vi "Check Data Model.vi"(8 "error in":errorcluster, 11 "device data model in":refnum<class "Standard Data Model.lvclass">) -> (0 "error out":errorcluster, 3 "device data model out":refnum<class "Standard Data Model.lvclass">)   [LabVIEW 2012, in "Standard Data Model.lvclass"]
doc: "This VI ensures that the data model has at least 65,535 values of every type. This is required for certain modbus function codes."
uses:
  Standard Data Model.lvclass
  Standard Data Model.lvclass/Standard Data Model.ctl
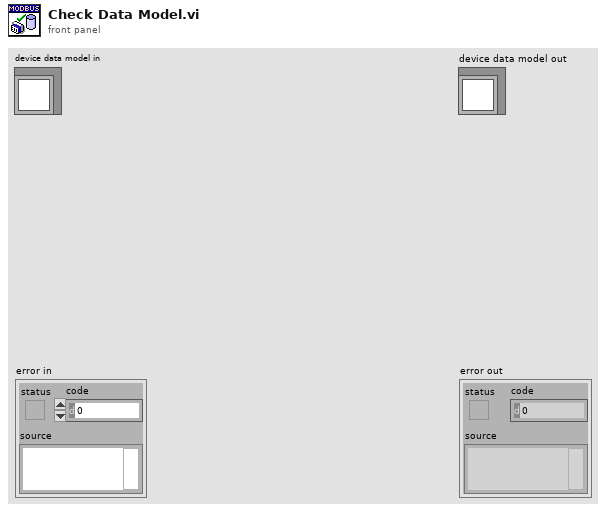
[diagram p1: front panel]
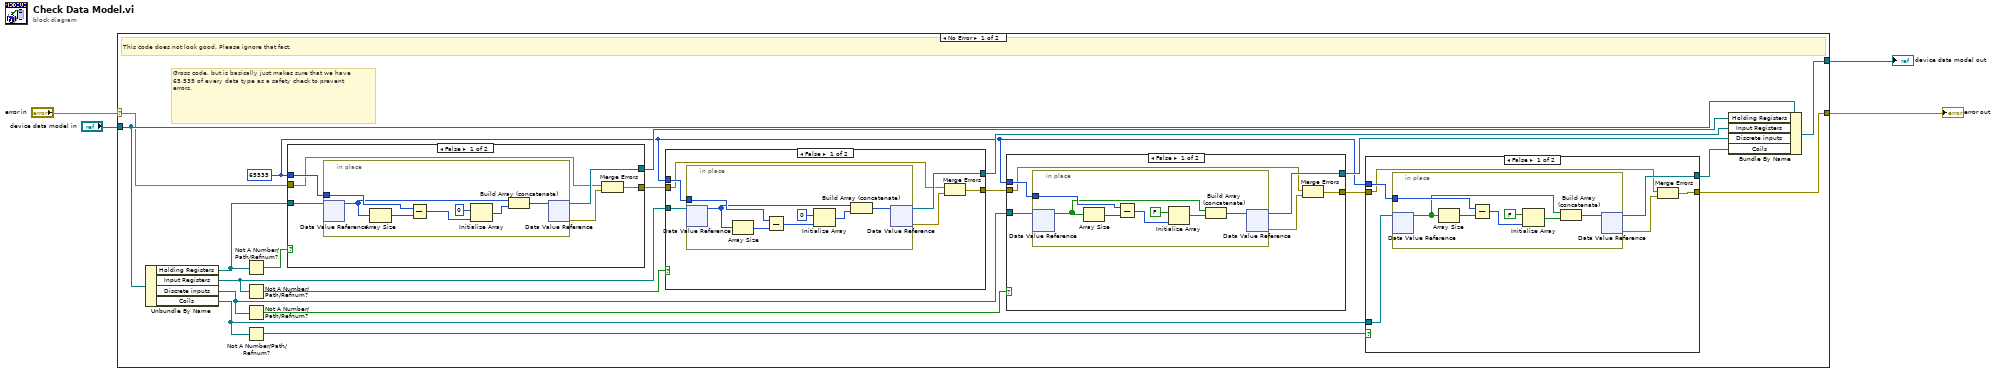
[diagram p0: block diagram]
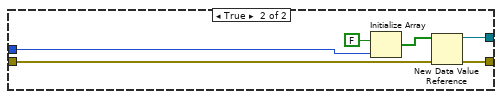
[diagram p2: hidden frame]
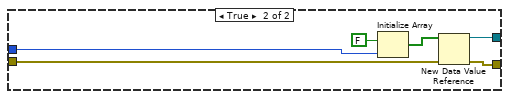
[diagram p3: hidden frame]
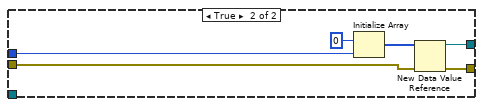
[diagram p4: hidden frame]
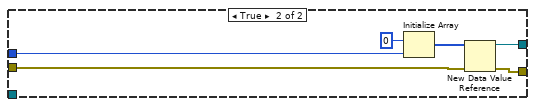
[diagram p5: hidden frame]
diagram:
  n1 = case shown="No Error" "error in" {
    selector: "error in" -> [w5 w102]
    tunnel: "device data model in" -> [w19 w101]
    tunnel: [w18 w101] -> w3
    tunnel: [w9 w102] -> w2
    frame No Error {
      w6 = u16 65535 ("x")
      # "Gross code, but is basically just makes sure that we have 65,535 of every data type as a safety check to prevent errors."
      # "This code does not look good. Please ignore that fact."
      n2 = Unbundle By Name(w19) -> ("Holding Registers"=w23:refnum<data-value>, "Input Registers"=w21:refnum<data-value>, "Discrete inputs"=w14:refnum<data-value>, "Coils"=w7:refnum<data-value>)
      n3 = Not A Number/Path/Refnum?(number/path/refnum=w23) -> (NaN/Path/Refnum?=w24:bool)
      n4 = Not A Number/Path/Refnum?(number/path/refnum=w21) -> (NaN/Path/Refnum?=w22:bool)
      n5 = Not A Number/Path/Refnum?(number/path/refnum=w14) -> (NaN/Path/Refnum?=w15:bool)
      n6 = Not A Number/Path/Refnum?(number/path/refnum=w7) -> (NaN/Path/Refnum?=w11:bool)
      n7 = case shown="False" w24 {
        tunnel: w5 -> [w82 w99]
        tunnel: [w84 w97] -> w17
        tunnel: [w85 w96] -> w20
        tunnel: w23 -> [w86 _]
        tunnel: w6 -> [w83 w95]
        frame False {
          n8 = in-place {
            in-place-border: w83 -> [w94]
            n9 = in-place-dvr #1(w86) -> (w90:u16[])  [unwired: 1 out]
            n10 = Array Size(array=w90) -> (size(s)=w93:i32)
            n11 = Subtract(x=w94, y=w93) -> (x-y=w92:i32)
            n12 = Initialize Array(u16 0 ("element"), w92) -> (w89:u16[])
            n13 = Build Array (concatenate)(w90, w89) -> (w88:u16[])
            n14 = in-place-dvr #1(w88) -> (w84:refnum<data-value>, w87:errorcluster)
          }
          n15 = Merge Errors(w82, w87) -> (w85:errorcluster)
        }
        frame True {
          n16 = Initialize Array(u16 0 ("element"), w95) -> (w98:u16[])
          n17 = New Data Value Reference(data value=w98, error in=w99) -> (data value reference=w97:refnum<data-value>, error out=w96:errorcluster)
        }
      }
      n18 = case shown="False" w22 {
        tunnel: w20 -> [w63 w80]
        tunnel: [w65 w78] -> w16
        tunnel: [w66 w77] -> w12
        tunnel: w21 -> [w67 _]
        tunnel: w6 -> [w64 w76]
        frame False {
          n19 = in-place {
            in-place-border: w64 -> [w75]
            n20 = in-place-dvr #2(w67) -> (w71:u16[])  [unwired: 1 out]
            n21 = Array Size(array=w71) -> (size(s)=w74:i32)
            n22 = Subtract(x=w75, y=w74) -> (x-y=w73:i32)
            n23 = Initialize Array(u16 0 ("element"), w73) -> (w70:u16[])
            n24 = Build Array (concatenate)(w71, w70) -> (w69:u16[])
            n25 = in-place-dvr #2(w69) -> (w65:refnum<data-value>, w68:errorcluster)
          }
          n26 = Merge Errors(w63, w68) -> (w66:errorcluster)
        }
        frame True {
          n27 = Initialize Array(u16 0 ("element"), w76) -> (w79:u16[])
          n28 = New Data Value Reference(data value=w79, error in=w80) -> (data value reference=w78:refnum<data-value>, error out=w77:errorcluster)
        }
      }
      n29 = case shown="False" w15 {
        tunnel: w12 -> [w44 w62]
        tunnel: [w46 w57] -> w13
        tunnel: [w47 w60] -> w8
        tunnel: w14 -> [w48 _]
        tunnel: w6 -> [w45 w59]
        frame False {
          n30 = in-place {
            in-place-border: w45 -> [w56]
            n31 = in-place-dvr #3(w48) -> (w52:bool[])  [unwired: 1 out]
            n32 = Array Size(array=w52) -> (size(s)=w55:i32)
            n33 = Subtract(x=w56, y=w55) -> (x-y=w54:i32)
            n34 = Initialize Array(FALSE, w54) -> (w51:bool[])
            n35 = Build Array (concatenate)(w52, w51) -> (w50:bool[])
            n36 = in-place-dvr #3(w50) -> (w46:refnum<data-value>, w49:errorcluster)
          }
          n37 = Merge Errors(w44, w49) -> (w47:errorcluster)
        }
        frame True {
          n38 = Initialize Array(FALSE, w59) -> (w61:bool[])
          n39 = New Data Value Reference(data value=w61, error in=w62) -> (data value reference=w57:refnum<data-value>, error out=w60:errorcluster)
        }
      }
      n40 = case shown="False" w11 {
        tunnel: w8 -> [w25 w43]
        tunnel: [w27 w39] -> w10
        tunnel: [w28 w41] -> w9
        tunnel: w7 -> [w29 _]
        tunnel: w6 -> [w26 w40]
        frame False {
          n41 = in-place {
            in-place-border: w26 -> [w37]
            n42 = in-place-dvr #4(w29) -> (w33:bool[])  [unwired: 1 out]
            n43 = Array Size(array=w33) -> (size(s)=w36:i32)
            n44 = Subtract(x=w37, y=w36) -> (x-y=w35:i32)
            n45 = Initialize Array(FALSE, w35) -> (w32:bool[])
            n46 = Build Array (concatenate)(w33, w32) -> (w31:bool[])
            n47 = in-place-dvr #4(w31) -> (w27:refnum<data-value>, w30:errorcluster)
          }
          n48 = Merge Errors(w25, w30) -> (w28:errorcluster)
        }
        frame True {
          n49 = Initialize Array(FALSE, w40) -> (w42:bool[])
          n50 = New Data Value Reference(data value=w42, error in=w43) -> (data value reference=w39:refnum<data-value>, error out=w41:errorcluster)
        }
      }
      n51 = Bundle By Name(cluster=w19, "Holding Registers"=w17, "Input Registers"=w16, "Discrete inputs"=w13, "Coils"=w10) -> (w18:refnum<class "Standard Data Model.lvclass">)
    }
    frame Error {
    }
  }
  "error out" <- w2
  "device data model out" <- w3
